vi "data array refresh.vi"(8 "error in (no error)":errorcluster, 11 "queue out":refnum<queue>) -> ()   [LabVIEW 2021]
panel:
  out "Array":dbl[][](array[numeric])
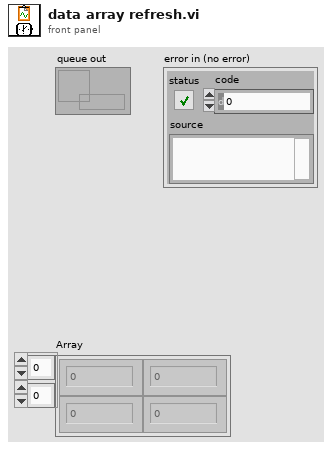
[diagram p1: front panel]
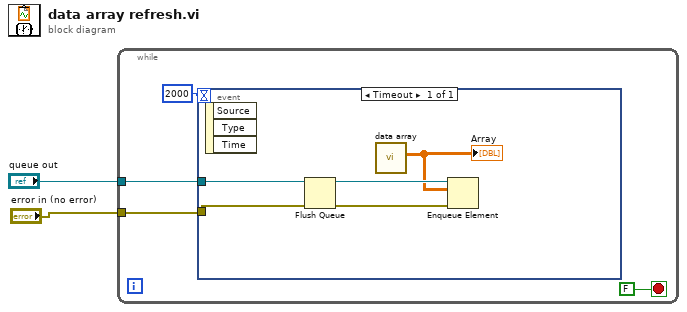
[diagram p0: block diagram]
diagram:
  n1 = while {
    tunnel: "queue out" -> [w3]
    tunnel: "error in (no error)" -> [w4]
    stop <- FALSE stop-if-true
    n2 = event shown="[0] Timeout" {
      selector: _ -> [_]
      dyn-events: _ -> [_]
      timeout: 2000 -> [_]
      tunnel: w3 -> [w8]
      tunnel: w4 -> [w7]
      event Timeout {
        n3 = event-data() -> ()  [unwired: 1 in, 3 out]
        n4 = Flush Queue(queue=w8, error in (no error)=w7) -> (queue out=w11:refnum<queue>, error out=w10:errorcluster)  [unwired: 1 out]
        n5 = call "data array.vi"() -> ("Array"=w9:dbl[][])  [unwired: 11 in]
        "Array" <- w9
        n6 = Enqueue Element(queue=w11, element=w9, error in (no error)=w10) -> ()  [unwired: 1 in, 3 out]
      }
    }
  }
